vi "TEST - Error 1403 on Cluster of Array.vi"() -> ()   [LabVIEW 2020, in "TEST - JKI JSON Object Serialization.lvlib"]
uses:
  TEST - JKI JSON Object Serialization.lvlib
  array-in-a-cluster.lvclass
  <vilib>/addons/_JKI Toolkits/Caraya/classes/Test/Test.lvclass
  source/library/JKI JSON Object Serialization.lvlib
  <vilib>/addons/_JKI Toolkits/Caraya/classes/Assert/Assert.lvclass
panel:
  out "error out":errorcluster
  in  "error in":errorcluster
  out "JSON String":string
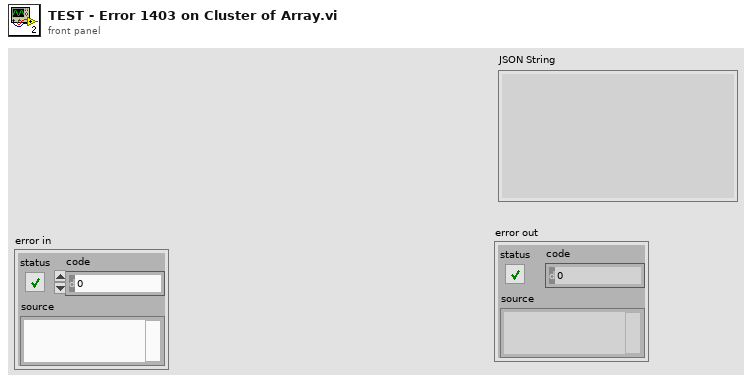
[diagram p1: front panel]
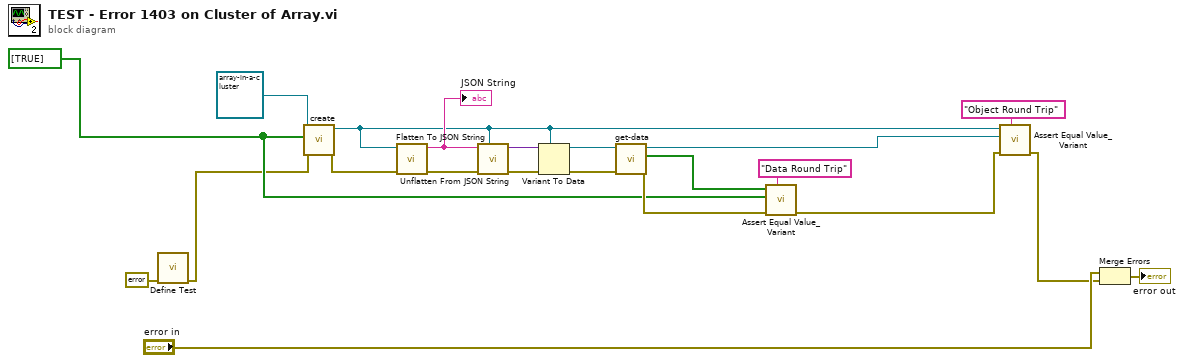
[diagram p0: block diagram]
diagram:
  w3 = bool[] [TRUE] ("Cluster.Array")
  n1 = call <vilib>:"Define Test.vi"("error in (no error)"=errorcluster {"status"=FALSE, "code"=0, "source"=""}) -> ("error out"=w2:errorcluster)  [unwired: 9 in, 1 out]
  n2 = call "create.vi"("error in (no error)"=w2, "Cluster.Array"=w3, "tempy in"=refnum<class "array-in-a-cluster.lvclass"> refnum) -> ("error out"=w1:errorcluster, "tempy out"=w10:refnum<class "array-in-a-cluster.lvclass">)  [unwired: 7 in]
  n3 = call "Flatten To JSON String.vi"("error in (no error)"=w1, "Variant"=w10) -> ("error out"=w17:errorcluster, "JSON String"=w18:string)  [unwired: 8 in]
  "JSON String" <- w18
  n4 = call "Unflatten From JSON String.vi"("Type and Defaults"=w10, "error in (no error)"=w17, "JSON String"=w18) -> ("error out"=w16:errorcluster, "Variant"=w15:variant)  [unwired: 7 in]
  n5 = Variant To Data(error in=w16, type=w10, Variant=w15) -> (data=w8:refnum<class "array-in-a-cluster.lvclass">, error out=w7:errorcluster)
  n6 = call "get-data.vi"("error in (no error)"=w7, "tempy in"=w8) -> ("error out"=w4:errorcluster, "Cluster.Array"=w5:bool[], "tempy out"=w6:refnum<class "array-in-a-cluster.lvclass">)  [unwired: 7 in]
  n7 = call <vilib>:"Assert Equal Value_Variant.vi"("Label"="Data Round Trip", "error in (no error)"=w4, "Y"=w3, "X"=w5) -> ("error out"=w14:errorcluster)  [unwired: 6 in, 1 out]
  n8 = call <vilib>:"Assert Equal Value_Variant.vi"("Label"="Object Round Trip", "error in (no error)"=w14, "Y"=w6, "X"=w10) -> ("error out"=w13:errorcluster)  [unwired: 6 in, 1 out]
  n9 = Merge Errors("error in", w13) -> (→"error out":errorcluster)
